vi "VPA QC PSetPt FGV.vi"(8 "error in (no error)":errorcluster, 9 "Function":enum16{"R", "W"}(ring), 10 "PSetPt In":u32=100 min=100) -> (0 "error out":errorcluster, 2 "PSetPt Out":u32=100)   [LabVIEW 2013]
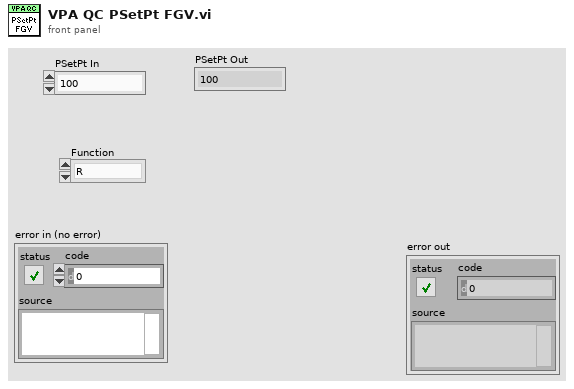
[diagram p1: front panel]
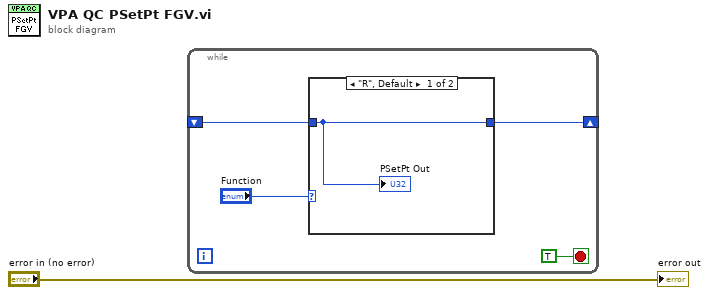
[diagram p0: block diagram]
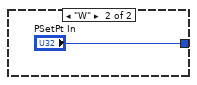
[diagram p2: hidden frame]
diagram:
  n1 = while {
    shift-right: [w3] -> _
    shift-left: _ -> [w2]
    stop <- TRUE stop-if-true
    n2 = case shown="\"R\", Default" "Function" {
      tunnel: [w6 "PSetPt In"] -> w3
      tunnel: w2 -> [w6 _]
      frame "R", Default {
        "PSetPt Out" <- w6
      }
      frame "W" {
      }
    }
  }
  "error out" <- "error in (no error)"
